vi "Actor Core.vi"(8 "error in":errorcluster, 11 "Normal Active Station Time Remaining View In":refnum<class "Normal Active Option Elapsed Time View.lvclass">) -> (0 "error out":errorcluster, 3 "Actor out":refnum<class "Actor.lvclass">)   [LabVIEW 2019, in "Normal Active Option Elapsed Time View.lvclass"]
doc: "(<B>Filename</B>: Actor Framework.lvlib:Actor.lvclass:Actor Core.vi)\n\nReceives messages to the actor, reacts to them, and initiates any error handling that may shut the actor down.\n\nDescendant classes may override this VI to append parallel tasks for the actor to complete while it handles messages. Overrides use the Call Parent Method node.\n\n<License>\nCopyright © 2017 Composed Systems, LLC | All rights reserved\nwww.composed.io\n\nAuthor: Ethan Stern <ethan.stern@composed.io>\n\nThis software is provided \"AS IS\" WITHOUT WARRANTIES, either express or implied, AND IS FOR EDUCATIONAL PURPOSES ONLY.\n</License>"
uses:
  <vilib>/gpm_packages/@cs/Car-wash/Source/Normal Active Station Time Remaining View/Normal Active Station Time Remaining View/Normal Active Option Elapsed Time View.lvclass
  <vilib>/gpm_packages/@cs/Car-wash/Source/Active Station Time Remaining View Definition/Active Station Time Remaining View Definition/Active Option Elapsed Time View Definition.lvclass
  C:/Program Files/National Instruments/LabVIEW 2019/vi.lib/gpm_packages/@cs/composed-car-wash/Source/Active Station Time Remaining View Definition/Active Station Time Remaining View Definition/Active Option Elapsed Time View Definition.lvclass
  C:/Program Files/National Instruments/LabVIEW 2019/vi.lib/gpm_packages/@cs/mva-viewable/Source/IViewable/IViewable/IViewable.lvclass
  C:/Program Files/National Instruments/LabVIEW 2019/vi.lib/gpm_packages/@cs/mva-viewable/Source/ActorEvents/IEventAggregator/IEventAggregator.lvclass
  C:/Program Files/National Instruments/LabVIEW 2019/vi.lib/gpm_packages/@cs/mva-core/Source/IObserver/IObserver/IObserver.lvclass
  C:/Program Files/National Instruments/LabVIEW 2019/vi.lib/ActorFramework/Actor/Actor.lvclass
  <vilib>/ActorFramework/Actor/Actor.lvclass
panel:
  out "Elapsed Time":dbl format="%0.2f"
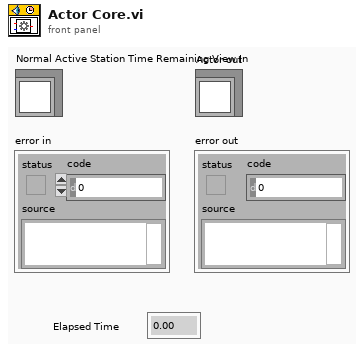
[diagram p1: front panel]
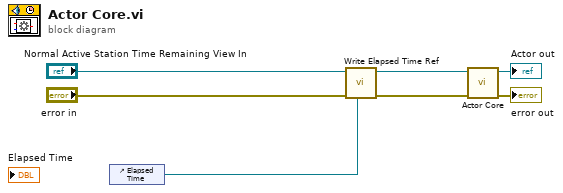
[diagram p0: block diagram]
diagram:
  n1 = control-ref of="Elapsed Time"() -> (w1:refnum<vi>)
  n2 = call <vilib>:"Write Elapsed Time Ref.vi"("Elapsed Time Ref"=w1, "Active Station Time Remaining View Definition in"="Normal Active Station Time Remaining View In") -> ("Active Station Time Remaining View Definition out"=w2:refnum<class "Normal Active Option Elapsed Time View.lvclass">)  [unwired: 9 in]
  n3 = call-parent "Actor Core.vi"("error in"="error in", "Active Station Time Remaining View Definition In"=w2) -> ("error out"=→"error out":errorcluster, "Actor out"=→"Actor out":refnum<class "Actor.lvclass">)  [unwired: 8 in]
